vi "Find Device.vi"(8 "error in":errorcluster, 11 "6509 in":refnum<class "6509.lvclass">) -> (0 "error out":errorcluster, 3 "6509 out":refnum<class "6509.lvclass">)   [LabVIEW 2019, in "6509.lvlib" / "6509.lvclass"]
uses:
  Library/6509.lvclass
  C:/Users/Public/Documents/Development/builds/Instruments/Instruments.lvlibp/Library/Instruments.lvclass
  Library/6509.lvclass/6509.ctl
  builds/Instruments/Instruments.lvlibp/Accessors/Read Resource.vi
  <resource>/objmgr/daqmx.rc
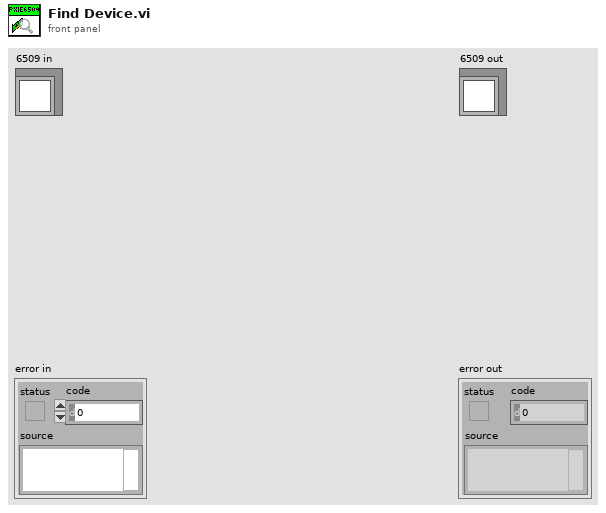
[diagram p1: front panel]
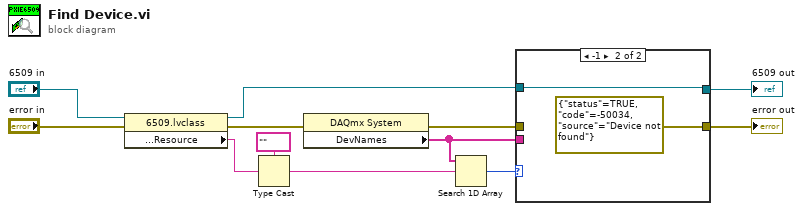
[diagram p0: block diagram]
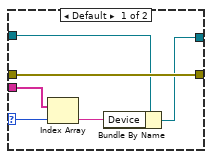
[diagram p2: hidden frame]
diagram:
  n1 = property class="6509.lvclass"(reference="6509 in", error in="error in") -> (reference out=w2:refnum<class "6509.lvclass">, error out=w9:errorcluster, "Accessors:Configuration:Resource"=w10:string)
  n2 = Type Cast(type=tag "" ("DAQmx Device Name"), x=w10) -> (*(type *) &x=w8:tag)
  n3 = property class="DAQmx System"(error in=w9) -> (error out=w5:errorcluster, "DevNames"=w6:tag[])  [unwired: 1 in, 1 out]
  n4 = Search 1D Array(1D array=w6, element=w8) -> (index of element=w7:i32)  [unwired: 1 in]
  n5 = case shown="-1" w7 {
    selector: w7 -> [w17 _]
    tunnel: w6 -> [w18 _]
    tunnel: w5 -> [w16 _]
    tunnel: [w16 errorcluster {"status"=TRUE, "code"=-50034, "source"="Device not found"} ("error out")] -> w4
    tunnel: w2 -> [w15 w20]
    tunnel: [w13 w20] -> w1
    frame Default {
      n6 = Index Array(array=w18, index=w17) -> (element=w14:tag)
      n7 = Bundle By Name(cluster=w15, "Device"=w14) -> (w13:refnum<class "6509.lvclass">)
    }
    frame -1 {
    }
  }
  "error out" <- w4
  "6509 out" <- w1
